vi "Connect and Start Tasks.vi"(8 "error in":errorcluster, 11 "CRDS in":refnum<class "CRDS.lvclass">=refnum) -> (0 "error out":errorcluster, 3 "CRDS out":refnum<class "CRDS.lvclass">)   [LabVIEW 2012, in "CRDS.lvclass"]
doc: "Connect the counter internal output of the YAG to the PXI Trig0 on the backplane and then start all tasks."
uses:
  CRDS.lvclass
  <resource>/objmgr/daqmx.rc
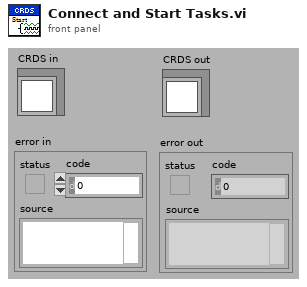
[diagram p1: front panel]
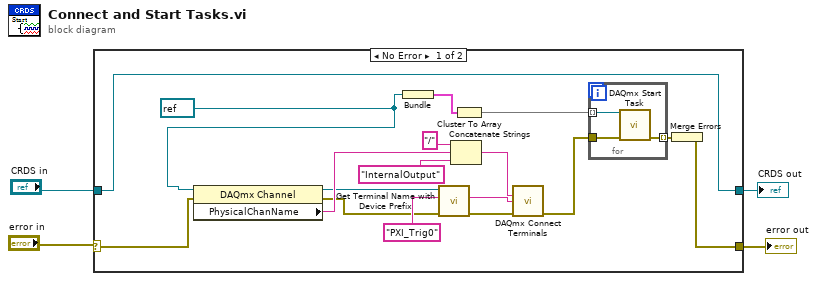
[diagram p0: block diagram]
diagram:
  n1 = case shown="No Error" "error in" {
    selector: "error in" -> [w9 w26]
    tunnel: [w13 w26] -> w3
    tunnel: [w12 w25] -> w1
    tunnel: "CRDS in" -> [w12 w25]
    frame No Error {
      w5 = refnum<k21> refnum ("task/channels in")
      n2 = property class="DAQmx Channel"(reference=w5, error in=w9) -> (reference out=w10:refnum<k21>, error out=w8:errorcluster, "PhysicalChanName"=w11:tag)
      n3 = Bundle("task/channels in"=w5) -> (w6:cluster{"task/channels in":refnum<k21>})  [unwired: 1 in]
      n4 = call "Get Terminal Name with Device Prefix.vi"("error in (no error)"=w8, "Local Terminal Name"="PXI_Trig0", "task/channels in"=w10) -> ("error out"=w19:errorcluster, "Terminal Name with Device Prefix"=w17:tag)  [unwired: 6 in, 1 out]
      n5 = Concatenate Strings("/", w11, "InternalOutput" ("string")) -> (w16:string)
      n6 = Cluster To Array(cluster=w6) -> (array=w7:refnum<k21>[])
      n7 = call <vilib>:"DAQmx Connect Terminals.vi"("source terminal"=w16, "destination terminal"=w17, "error in"=w19) -> ("error out"=w15:errorcluster)  [unwired: 12 in]
      n8 = for {
        tunnel: w7 -> [w24] mode=indexing
        tunnel: w15 -> [w23]
        tunnel: [w22] -> w14 mode=indexing
        n9 = call <vilib>:"DAQmx Start Task.vi"("task/channels in"=w24, "error in"=w23) -> ("error out"=w22:errorcluster)  [unwired: 12 in, 1 out]
      }
      n10 = Merge Errors(w14) -> (w13:errorcluster)
    }
    frame Error {
    }
  }
  "error out" <- w3
  "CRDS out" <- w1
